vi "Get RT Image Metadata.vi"(8 "error in (no error)":errorcluster) -> (0 "error out":errorcluster, 3 "RT Image Metadata":T1)   [LabVIEW 2020]
doc: "This VI reads the current image properties and sends them to the telemetry handler."
uses:
  Type Definitions/RT Image Metadata.ctl
  Type Definitions/Enum - Metadata.ctl
  Type Definitions/Payload Class.ctl
  <resource>/objmgr/nisysapi.rc
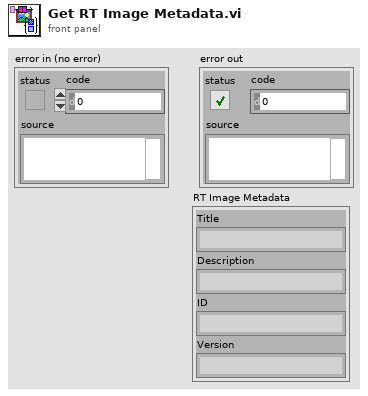
[diagram p1: front panel]
types:
  T1 = typedef "RT Image Metadata.ctl" = cluster{"Title":string, "Description":string, "ID":string, "Version":string}
  T2 = typedef "Payload Class.ctl" = enum16{"System State", "Parameters", "Metadata", "Software Monitor", "Data", "Commands"}
  T3 = typedef "Enum - Metadata.ctl" = enum16{"Computer Metadata", "Computer Resources", "RT Image Metadata", "Startup Settings", "Telemetry Recorder Status"}
  T4 = typedef "System Resources.ctl" = cluster{"System Session":refnum<k21>, "System Resource":refnum<k20>, "FPGA VI Reference":refnum<k20>}
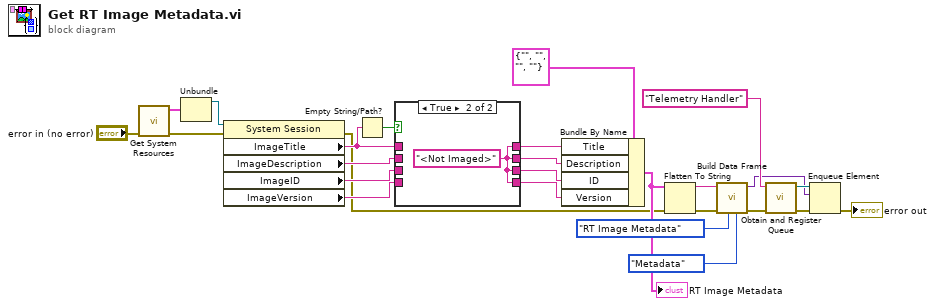
[diagram p0: block diagram]
diagram:
  n1 = call "Get System Resources.vi"("error in (no error)"="error in (no error)") -> ("error out"=w1:errorcluster, "System Resources"=w5:T4)  [unwired: 9 in]
  n2 = Unbundle(w5) -> ("System Session"=w3:refnum<k21>)  [unwired: 2 out]
  n3 = property class="System Session"(reference=w3, error in=w1) -> (error out=w4:errorcluster, "ImageTitle"=w20:string, "ImageDescription"=w22:string, "ImageID"=w23:string, "ImageVersion"=w26:string)  [unwired: 1 out]
  n4 = Empty String/Path?(string/path=w20) -> (empty?=w18:bool)
  n5 = case shown="True" w18 {
    tunnel: [w30 w31] -> w19
    tunnel: w20 -> [w30 _]
    tunnel: [w29 w31] -> w21
    tunnel: w22 -> [w29 _]
    tunnel: w23 -> [w28 _]
    tunnel: [w28 w31] -> w24
    tunnel: [w27 w31] -> w25
    tunnel: w26 -> [w27 _]
    frame False {
    }
    frame True {
      w31 = "<Not Imaged>" ("Image Metadata:Version")
    }
  }
  n6 = Bundle By Name(cluster=T1 {"Title"="", "Description"="", "ID"="", "Version"=""}, "Title"=w19, "Description"=w21, "ID"=w24, "Version"=w25) -> (w16:T1)
  "RT Image Metadata" <- w16
  n7 = Flatten To String(anything=w16, error in (no error)=w4) -> (data string=w15:string, error out=w12:errorcluster)  [unwired: 2 in, 1 out]
  n8 = call "Build Data Frame.vi"("Payload Class (Data)"=Payload_Class."Metadata", "Payload ID (0)"=Enum_-_Metadata."RT Image Metadata", "error in (no error)"=w12, "Payload (Empty String)"=w15) -> ("error out"=w8:errorcluster, "Frame"=w9:variant)  [unwired: 6 in]
  n9 = call "Obtain and Register Queue.vi"("error in (no error)"=w8, "name (unnamed)"="Telemetry Handler") -> ("error out"=w7:errorcluster, "Queue Out"=w10:refnum<queue>)  [unwired: 6 in, 2 out]
  n10 = Enqueue Element(queue=w10, element=w9, error in (no error)=w7) -> (error out=→"error out":errorcluster)  [unwired: 1 in, 2 out]
